vi "Create_Destination_for_Duplicate.vi"(8 "error in (no error)":errorcluster, 9 "subDirectory":string="data", 10 "Destinations in":refnum<class "AB_Destination.lvclass">[](array[class]), 11 "AB_Source in":refnum<class "AB_Source.lvclass">) -> (0 "error out":errorcluster, 1 "newPath":path, 2 "Destinations out":refnum<class "AB_Destination.lvclass">[](array[class]), 3 "AB_Source out":refnum<class "AB_Source.lvclass">)   [LabVIEW 2020, in "AB_Source.lvclass"]
uses:
  <vilib>/AppBuilder/AB_Classes/Source/AB_Source.lvclass
  <vilib>/AppBuilder/AB_Classes/Destination/AB_Destination.lvclass
  <vilib>/AppBuilder/AB_Classes/Source/AB_Source.lvclass/AB_Source.ctl
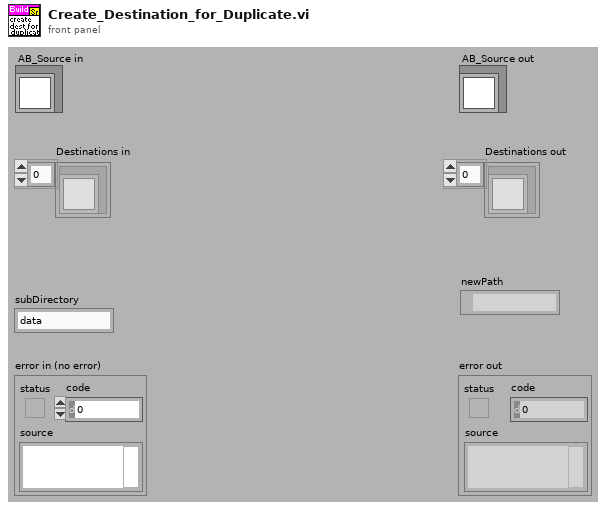
[diagram p1: front panel]
types:
  T1 = typedef "AB_Destination.ctl" = cluster{"destName":string, "path":path, "libraryName":string, "preserveHierarchy":bool, "eng_inBuild":bool, "eng_libraryReference":refnum<vi>, "eng_restictAddToNewLibrary":bool}
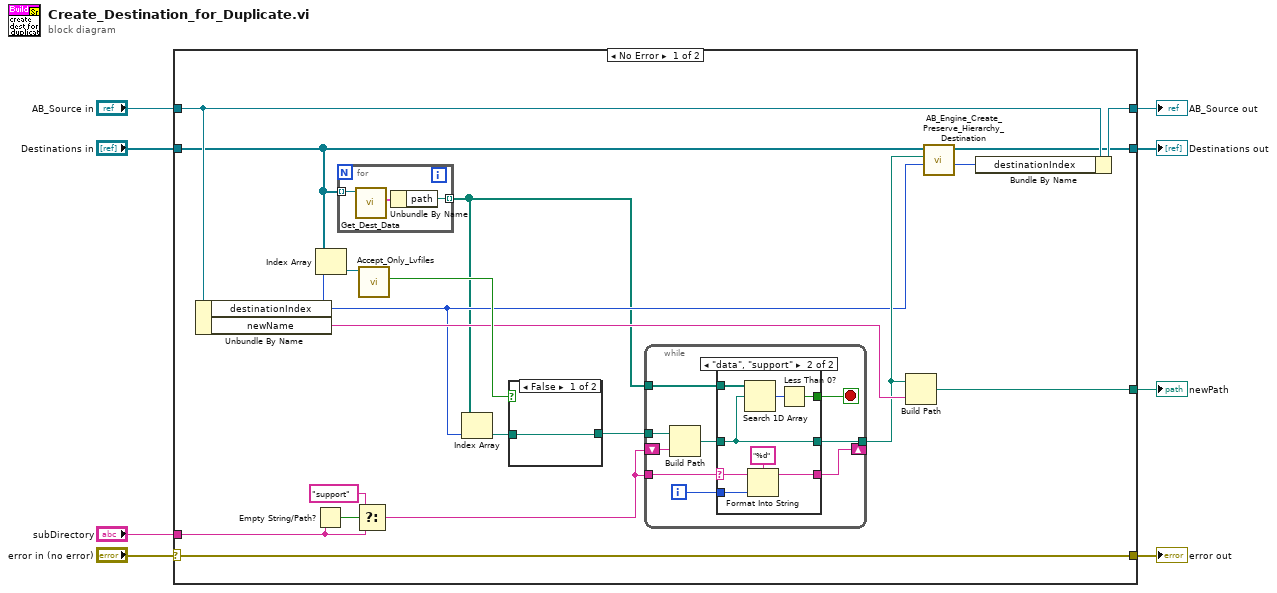
[diagram p0: block diagram]
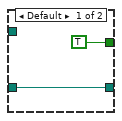
[diagram p2: hidden frame]
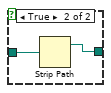
[diagram p3: hidden frame]
diagram:
  n1 = case shown="No Error" "error in (no error)" {
    selector: "error in (no error)" -> [w27 w55]
    tunnel: [w27 w55] -> w7
    tunnel: [w25 w54] -> w5
    tunnel: "AB_Source in" -> [w26 w54]
    tunnel: [w15 w53] -> w4
    tunnel: "Destinations in" -> [w14 w53]
    tunnel: [w21 _] -> w2
    tunnel: "subDirectory" -> [w20 _]
    frame No Error {
      n2 = Unbundle By Name(w26) -> ("destinationIndex"=w12:i32, "newName"=w22:string)
      n3 = Empty String/Path?(string/path=w20) -> (empty?=w19:bool)
      n4 = Index Array(array=w14, index=w12) -> (element=w13:refnum<class "AB_Destination.lvclass">)
      n5 = for {
        tunnel: w14 -> [w49] mode=indexing
        tunnel: [w47] -> w10 mode=indexing
        n6 = call <vilib>:"Get_Dest_Data.vi"("Class in"=w49) -> ("destName"=w48:T1)  [unwired: 1 in, 9 out]
        n7 = Unbundle By Name(w48) -> ("path"=w47:path)
      }
      n8 = Select(t="support", s=w19, f=w20) -> (s? t:f=w9:string)
      n9 = call-dynamic "Accept_Only_Lvfiles.vi"("AB_Destination in"=w13) -> ("onlyLVfiles"=w24:bool)  [unwired: 1 in, 9 out]
      n10 = Index Array(array=w10, index=w12) -> (element=w11:path)
      n11 = case shown="False" w24 {
        tunnel: w11 -> [w50 w52]
        tunnel: [w50 w51] -> w23
        frame False {
        }
        frame True {
          n12 = Strip Path(path=w52) -> (stripped path=w51:path)  [unwired: 1 out]
        }
      }
      n13 = while {
        tunnel: w23 -> [w36]
        tunnel: [w28] -> w16
        tunnel: w10 -> [w35]
        shift-right: [w31] -> _
        shift-left: w9 -> [w32]
        tunnel: w9 -> [w29]
        i -> [w33]
        stop <- w30 stop-if-true
        n14 = Build Path(base path=w36, name or relative path=w32) -> (appended path=w34:path)
        n15 = case shown="\"data\", \"support\"" w29 {
          selector: w29 -> [_ w40]
          tunnel: w35 -> [_ w46]
          tunnel: w34 -> [w37 w39]
          tunnel: w33 -> [_ w44]
          tunnel: [_ w43] -> w31
          tunnel: [TRUE w42] -> w30
          tunnel: [w37 w39] -> w28
          frame Default {
          }
          frame "data", "support" {
            n16 = Search 1D Array(1D array=w46, element=w39) -> (index of element=w41:i32)  [unwired: 1 out]
            n17 = Format Into String(format string="%d", initial string=w40, w44) -> (resulting string=w43:string)  [unwired: 1 in, 1 out]
            n18 = Less Than 0?(x=w41) -> (x < 0?=w42:bool)
          }
        }
      }
      n19 = Build Path(base path=w16, name or relative path=w22) -> (appended path=w21:path)
      n20 = call <vilib>:"AB_Engine_Create_Preserve_Hierarchy_Destination.vi"("parentIndex in"=w12, "newPath"=w16, "destinations in"=w14) -> ("destinationIndex out"=w17:i32, "destination out"=w15:refnum<class "AB_Destination.lvclass">[])  [unwired: 1 in, 6 out]
      n21 = Bundle By Name(cluster=w26, "destinationIndex"=w17) -> (w25:refnum<class "AB_Source.lvclass">)
    }
    frame Error {
    }
  }
  "error out" <- w7
  "AB_Source out" <- w5
  "Destinations out" <- w4
  "newPath" <- w2
